vi "bestMatch.vi"(10 "y":dbl, 11 "x":dbl) -> (2 "Y":dbl, 3 "X":dbl)   [LabVIEW 2018]
panel:
  out "i4":i32
  out "i3":i32
  out "i2":i32
  out "i1":i32
  out "px":dbl[](array[numeric])
  out "py":dbl[](array[numeric])
  out "cx":dbl[](array[numeric])
  out "cy":dbl[](array[numeric])
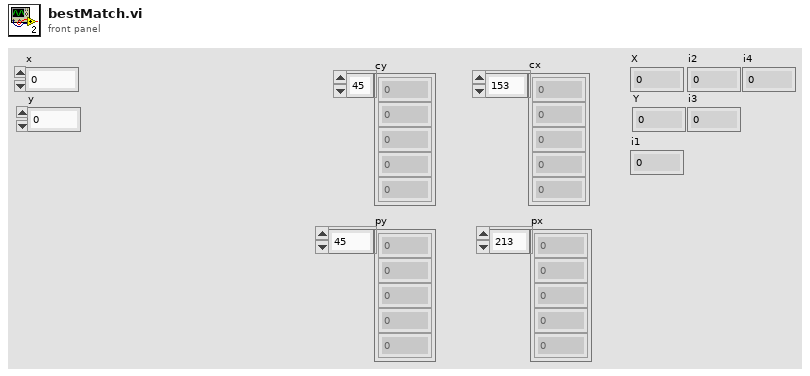
[diagram p1: front panel]
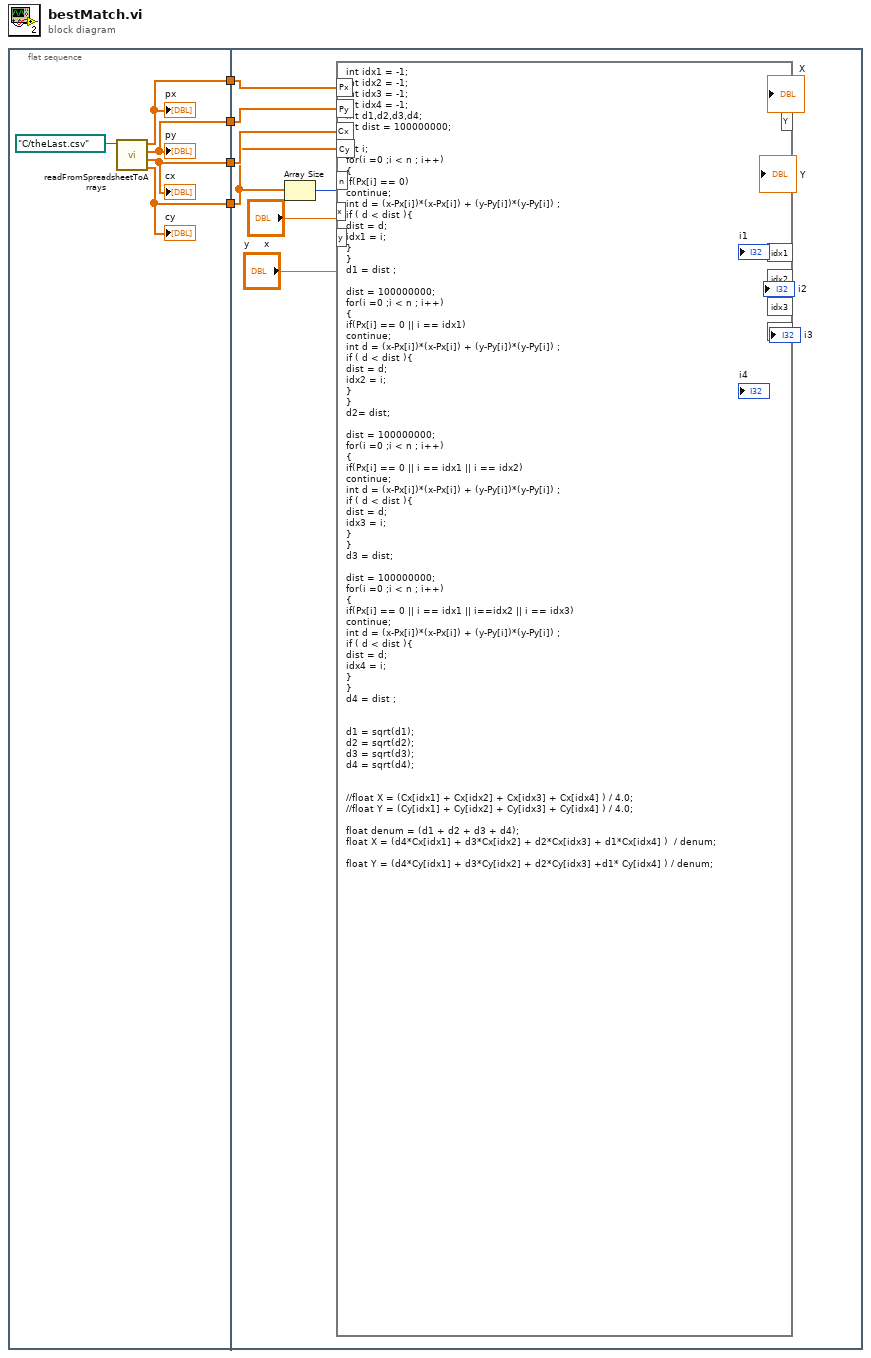
[diagram p0: block diagram]
diagram:
  n1 = flat-sequence {
    tunnel: [w8] -> w4
    tunnel: [w7] -> w3
    tunnel: [w6] -> w2
    tunnel: [w5] -> w1
    tunnel: w4 -> [w22]
    tunnel: w3 -> [w21]
    tunnel: w2 -> [w20]
    tunnel: w1 -> [w19]
    frame #0 {
      n2 = call "readFromSpreadsheetToArrays.vi"("file path (dialog if empty)"=path "C:/theLast.csv") -> ("column4"=w5:dbl[], "column3"=w6:dbl[], "column2"=w7:dbl[], "column1"=w8:dbl[])  [unwired: 7 in]
      "cy" <- w5
      "cx" <- w6
      "py" <- w7
      "px" <- w8
    }
    frame #1 {
      n3 = Array Size(array=w19) -> (size(s)=w18:i32)
      n4 = formula code="int idx1 = -1;\nint idx2 = -1;\nint idx3 = -1;\nint idx4 = -1;\nint d1,d2,d3,d4;\nint dist = 100000000;\n\nint i;\nfor(i =0 ;i < n ; i++)\n{\nif(Px[i] == 0)\ncontinue;\nint d = (x-Px[i])*(x-Px[i]) + (y-Py[i])*(y-Py[i]) ;\nif ( d < dist ){\ndist = d;\nidx1 = i;\n}\n}\nd1 = dist ;\n\ndist = 100000000;\nfor(i =0 ;i < n ; i++)\n{\nif(Px[i] == 0 || i == idx1)\ncontinue;\nint d = (x-Px[i])*(x-Px[i]) + (y-Py[i])*(y-Py[i]) ;\nif ( d < dist ){\ndist = d;\nidx2 = i;\n}\n}\nd2= dist;\n\ndist = 100000000;\nfor(i =0 ;i < n ; i++)\n{\nif(Px[i] == 0 || i == idx1 || i == idx2)\ncontinue;\nint d = (x-Px[i])*(x-Px[i]) + (y-Py[i])*(y-Py[i]) ;\nif ( d < dist ){\ndist = d;\nidx3 = i;\n}\n}\nd3 = dist;\n\ndist = 100000000;\nfor(i =0 ;i < n ; i++)\n{\nif(Px[i] == 0 || i == idx1 || i==idx2 || i == idx3)\ncontinue;\nint d = (x-Px[i])*(x-Px[i]) + (y-Py[i])*(y-Py[i]) ;\nif ( d < dist ){\ndist = d;\nidx4 = i;\n}\n}\nd4 = dist ;\n\n\nd1 = sqrt(d1);\nd2 = sqrt(d2);\nd3 = sqrt(d3);\nd4 = sqrt(d4);\n\n\n//float X = (Cx[idx1] + Cx[idx2] + Cx[idx3] + Cx[idx4] ) / 4.0;\n//float Y = (Cy[idx1] + Cy[idx2] + Cy[idx3] + Cy[idx4] ) / 4.0;\n\nfloat denum = (d1 + d2 + d3 + d4);\nfloat X = (d4*Cx[idx1] + d3*Cx[idx2] + d2*Cx[idx3] + d1*Cx[idx4] )  / denum;\n\nfloat Y = (d4*Cy[idx1] + d3*Cy[idx2] + d2*Cy[idx3] +d1* Cy[idx4] ) / denum;"("Px"=w22, "Py"=w21, "Cx"=w20, "Cy"=w19, "x"="x", "y"="y", "n"=w18) -> ("X"=→"X":dbl, "Y"=→"Y":dbl, "idx1"=→"i1":i32, "idx2"=→"i2":i32, "idx3"=→"i3":i32, "idx4"=→"i4":i32)
    }
  }
